vi "ecg_ncs_v1b.vi"() -> ()   [LabVIEW 2016]
uses:
  <instrlib>/niUSRP/niUSRP Timestamp.ctl
  C:/Program Files/National Instruments/LabVIEW 2016/examples/Instrument IO/Serial/support/Serial - Settings.ctl
  <vilib>/Analysis/coordinate.llb/Wrap Angle (array).vi
  <instrlib>/niUSRP/niUSRP Configure Time Start Trigger.vi
  <vilib>/Instr/_visa.llb/VISA Configure Serial Port (Instr).vi
  <instrlib>/niUSRP/niUSRP Write Tx Data (2D CDB).vi
  <instrlib>/niUSRP/niUSRP Fetch Rx Data (2D CDB).vi
  <vilib>/Analysis/3filter.llb/Butterworth Filter (DBL).vi
  <vilib>/measure/NI_MABase.lvlib
  <vilib>/Analysis/NI_AALBase.lvlib
  <vilib>/Analysis/NI_AALPro.lvlib
  <vilib>/Analysis/NI_AAL_Angle.lvlib
panel:
  out "Poor Sensor Quality: \nSensor off":bool
  out "Poor Sensor Quality: \nSensor on":bool
  out "Heart Rate 2":u16[](array[numeric])
  out "Stop Loop":bool
  out "Loop index":i32
  out "size(s)":i32
  in  "Read Count":u32=960
  out "return count":u32
  out "Serial Settings:Number of Bytes at Serial Port":u32
  in  "Serial Settings":T1={"baud rate"=57600, "data bits"=8, "parity"=enum."None", "stop bits"=10, "flow control"=0} {"flow control" items=["None"=0, "XON/XOFF"=1, "RTS/CTS"=2, "DTR/DSR"=4]; "stop bits" items=["1.0"=10, "1.5"=15, "2.0"=20]; "data bits" min=5 max=8 step=1; "baud rate" items=["75"=75, "110"=110, "134"=134, "150"=150, "300"=300, "600"=600, "1200"=1200, "1800"=1800, "2400"=2400, "4800"=4800, "7200"=7200, "9600"=9600, "14400"=14400, "19200"=19200, "28800"=28800, "38400"=38400, "56000"=56000, "57600"=57600, "115200"=115200, "128000"=128000, "230400"=230400]}
  in  "VISA resource name":refnum<visa-resource-name>="bmd101"
  in  "?":enum32{"ECG", "Heart Rate"}(tab)
  out "ECG":i16(graph)
  out "Heart Rate":u8[](graph)
  in  "Stop":bool
  in  "File Name":string="Test"
  in  "order1":i32=5
  in  "Path":path=path "D:/Research/SummerFall17Spring18/CnC/NCS/EcgNcsCorrelation"
  in  "Low-Pass Freq":dbl=200.0 format="%#_13g"
  in  "Sampling Rate":i32=500
  out "Gain":dbl=-15.0
  out "Bandwidth":dbl=56000000.0
  out "Coerced Carrier Frequency":dbl=2000000000.0 format="%#.17g"
  out "Coerced Tx IQ rate":dbl=1000000.0
  out "Coerced Rx IQ rate":dbl=1000000.0
  out "error IO":errorcluster={"status"=FALSE, "code"=-1074118647, "source"=""}
  in  "Rx Number of Samples":i32=20000
  in  "Tab Control 2":enum32{"NI-294x/295x", "NI-2900/2901"}(tab)=enum."NI-2900/2901"
  in  "channel 0 carrier\n frequency [Hz]":dbl=2000000000.0 format="%#_6p"
  in  "Rx carrier frequency [Hz]":dbl=2000000000.0 format="%#_6p"
  in  "Tx carrier frequency [Hz]":dbl=1000000000.0 format="%#_6p"
  in  "Start Trigger Time":T2={"whole seconds"=1, "fractional seconds"=0.0}
  out "Tx Active Antenna":string="TX1"
  in  "Tab Control":T3(tab)
  out "NCS tag Amp":dbl[](graph)=[0.013332788438327721, 0.0131552898712497, 0.012994905519721597, 0.012986271887777701, 0.013075284595455733, 0.013191204808537919, 0.013351894528100879, 0.01345386740636616, 0.013382234051438232, 0.013180163786137358]
  out "NCS tag Phase":dbl[](graph)=[114.08993023907641, 111.82225141412982, 110.02998222947944, 109.41153055749608, 110.12587965469353, 112.16042160734105, 113.81215100166591, 114.51260226782536, 113.6206368361215, 111.46787264294511]
  out "IQ":dbl[][](graph)
  out "Tag Amp":dbl[](graph)
  out "Tag Phase":dbl[](graph)
  out "Tx Waveform Graph":waveform(dbl)[](graph)=[{"t0"=timestamp(0 s since 1904-01-01), "dt"=1e-06, "Y"=array[2000 elements]}, {"t0"=timestamp(0 s since 1904-01-01), "dt"=1e-06, "Y"=array[2000 elements]}]
  in  "Channel 0\nTone Amplitude":dbl=0.707 step=0.05 format="%#.6g"
  in  "Channel 0 \nTone Frequency":dbl=5000.0 format="%#_6p"
  in  "Waveform Size":dbl=2000.0
  in  "Rx Active Antenna":string="RX2"
  in  "Device Name":refnum<k15>="MyB200"
  in  "Tx Gain":dbl=28.0 format="%#_6f"
  in  "Tx IQ Rate":dbl=1000000.0 format="%#_6p"
  in  "Rx Gain":dbl=32.0 format="%#_6f"
  in  "Rx IQ Rate":dbl=1000000.0 format="%#_6p"
  # "Rx Settings"
  # "Tx Settings"
  # "Note that on the NI-2900 and NI-2901, both Rx channels share an LO and both Tx channels share an LO. However, on the NI-294x/295x devices, Rx and Tx of channel 0 share an LO and Rx and Tx of channel 1 share an LO."
  # "This Tx graph should always have end and start tied up since this is being sent in a loop continuously. Otherwise phase jumps will be noticed."
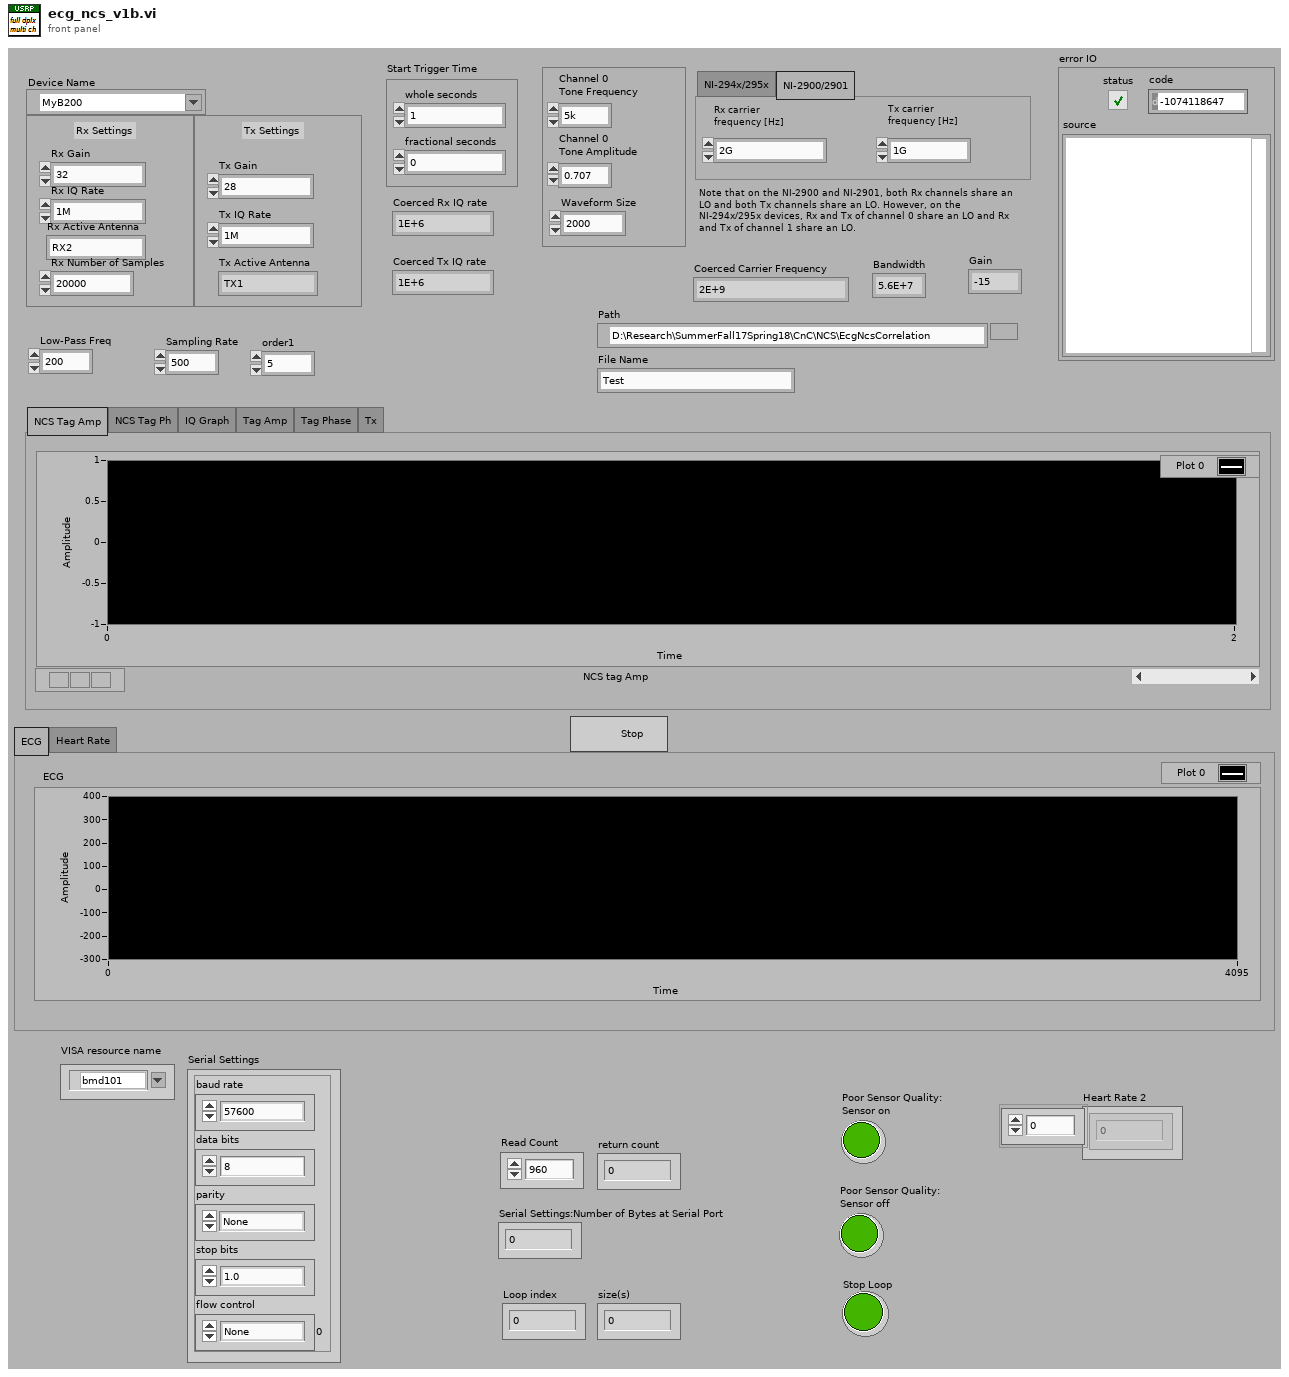
[diagram p1: front panel]
types:
  T1 = typedef "Serial - Settings.ctl" = cluster{"baud rate":u32, "data bits":u16, "parity":enum16{"None", "Odd", "Even", "Mark", "Space"}, "stop bits":u16, "flow control":u16}
  T2 = typedef "niUSRP Timestamp.ctl" = cluster{"whole seconds":u64, "fractional seconds":dbl}
  T3 = enum32{"NCS Tag Amp", "NCS Tag Ph", "IQ Graph", "Tag Amp", "Tag Phase", "Tx"}
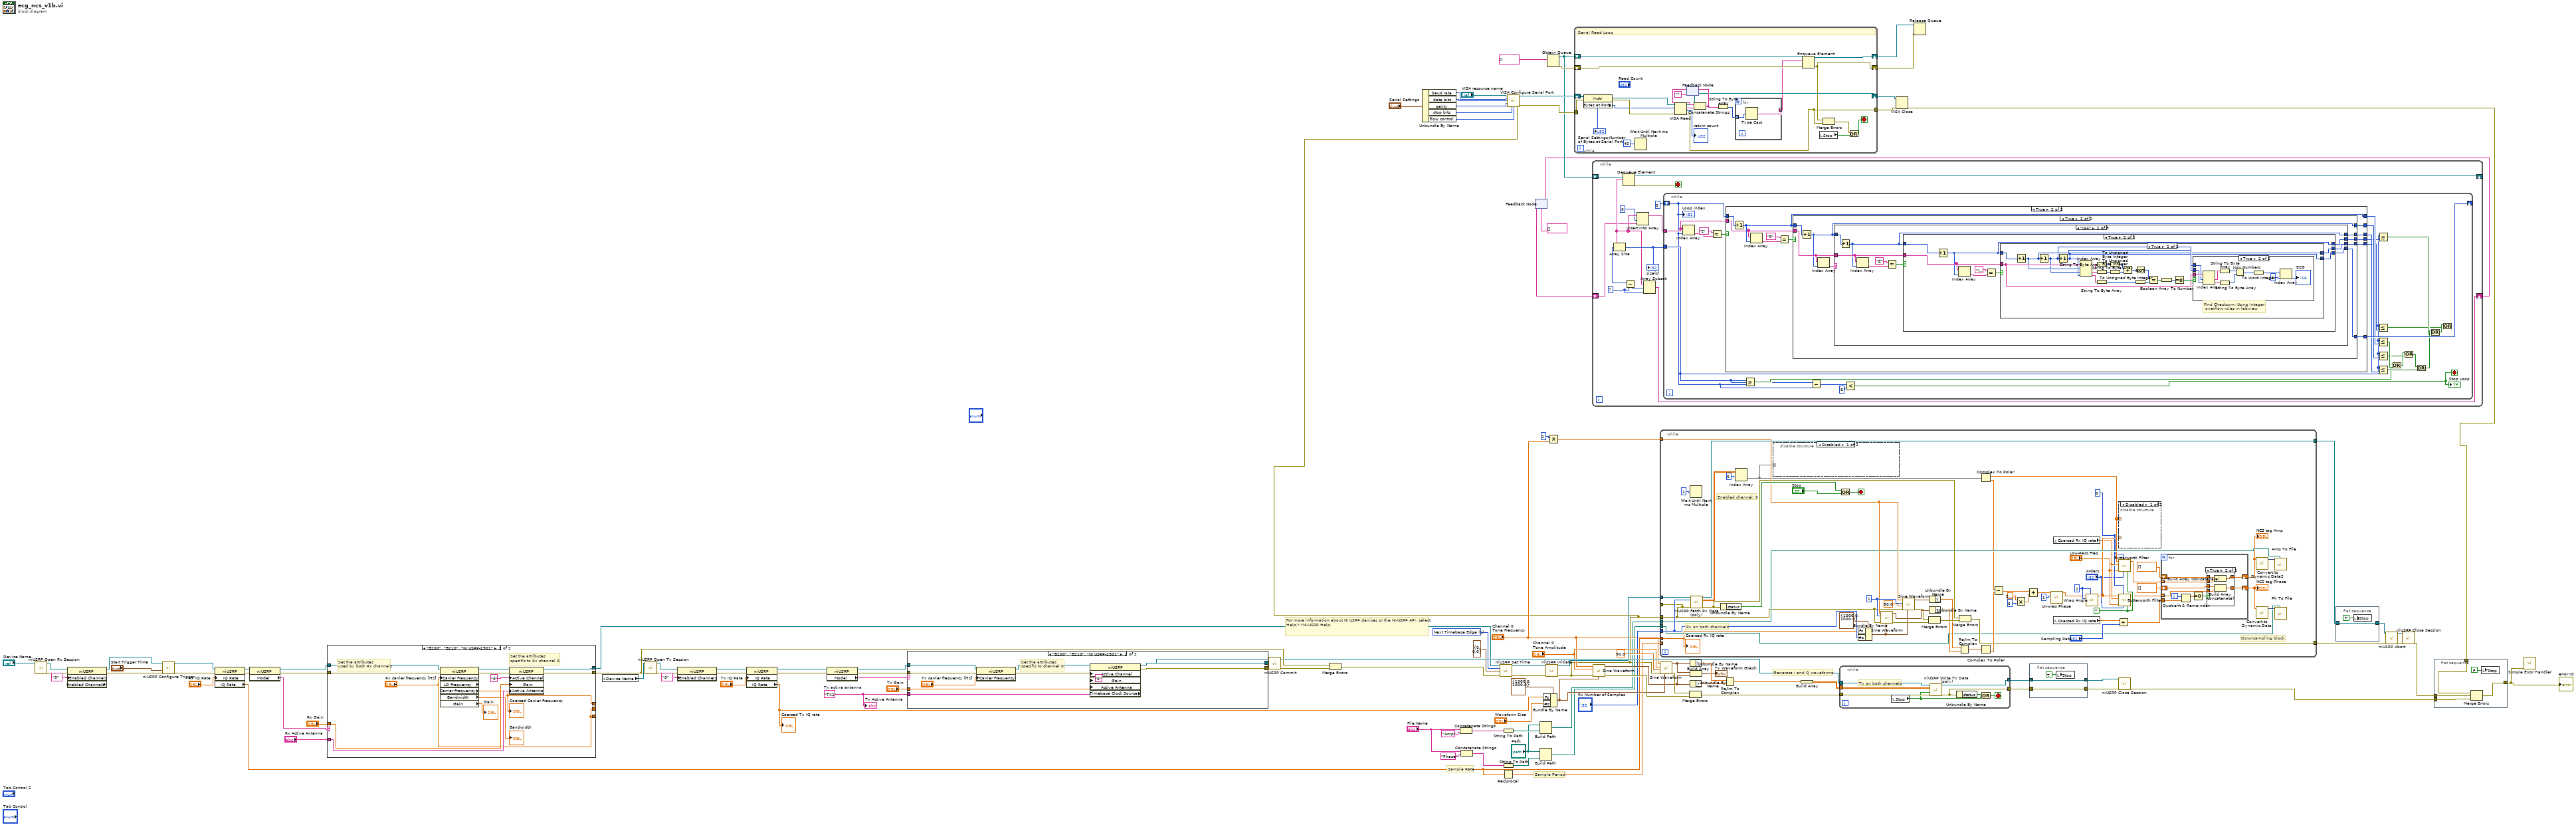
[diagram p0: block diagram]
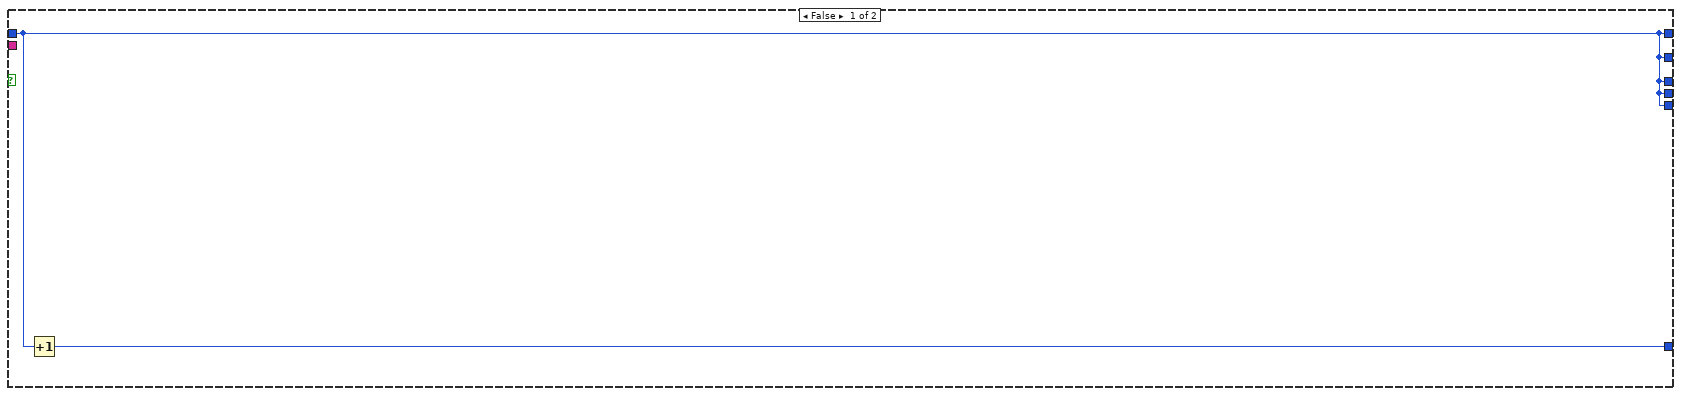
[diagram p2: hidden frame]
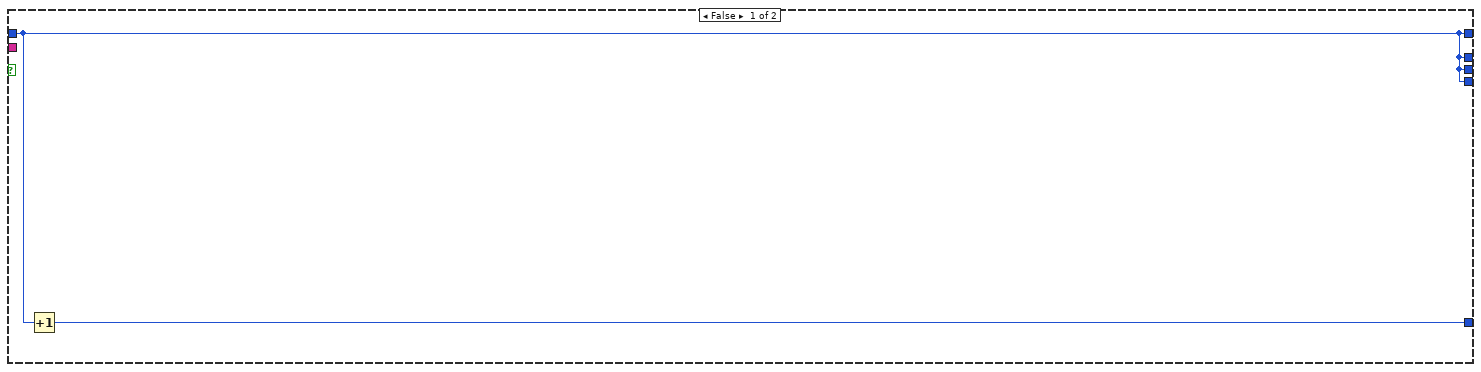
[diagram p3: hidden frame]
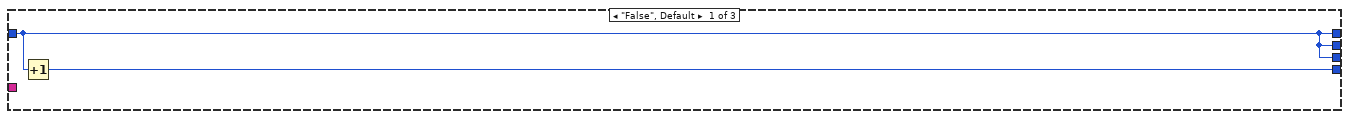
[diagram p4: hidden frame]
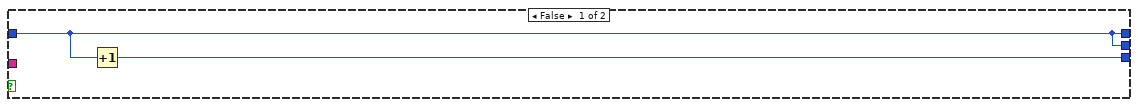
[diagram p5: hidden frame]
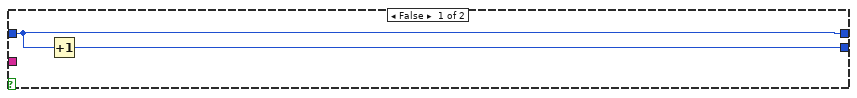
[diagram p6: hidden frame]
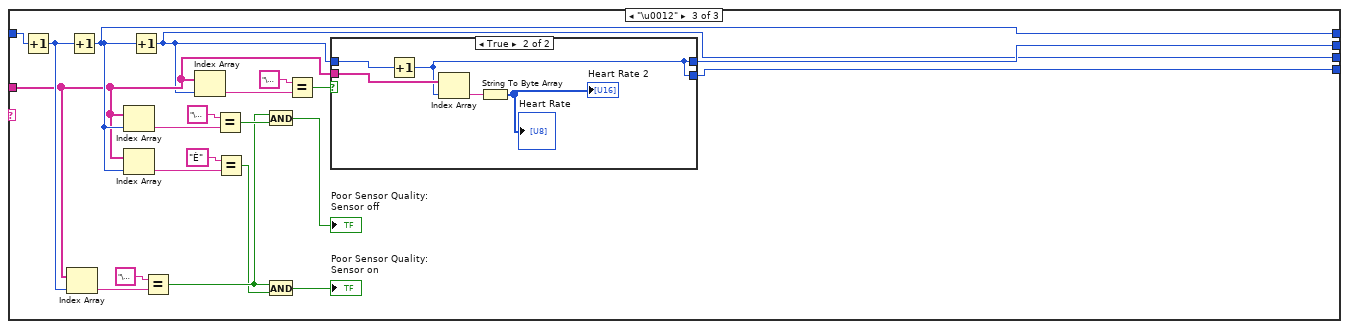
[diagram p8: hidden frame]
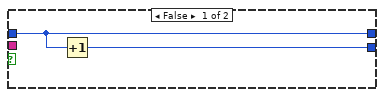
[diagram p9: hidden frame]
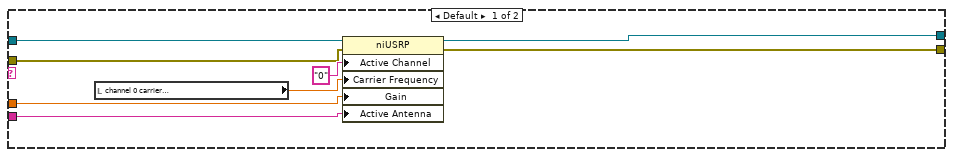
[diagram p10: hidden frame]
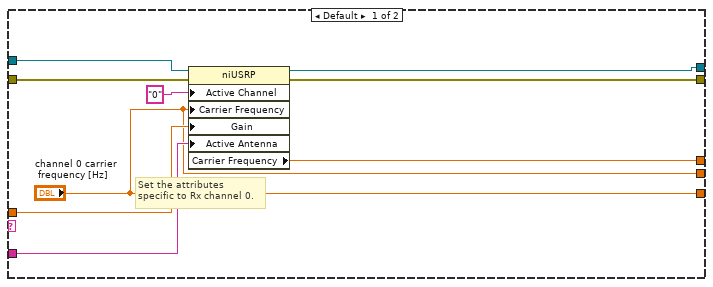
[diagram p11: hidden frame]
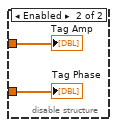
[diagram p12: hidden frame]
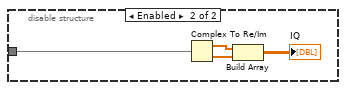
[diagram p13: hidden frame]
diagram:
  w81 = 1 items=["Now", "Next Timebase Edge"] ("apply timestamp")
  w50 = "TX1"  # Tx active antenna
  # "Sample Rate"
  # "Sample Period"
  # "For more information about NI USRP devices or the NI-USRP API, select Help>>NI-USRP Help."
  # "Generate I and Q waveforms."
  n1 = call <instrlib>:"niUSRP Open Rx Session.vi"("device names"="Device Name") -> ("session handle out"=w80:refnum<k15>, "error out"=w79:errorcluster)  [unwired: 13 in]
  n2 = property class="niUSRP" props=["Enabled Channels", "Enabled Channels"](reference=w80, error in=w79, "Enabled Channels"="0" ("Configuration:Enabled Channels")) -> (reference out=w78:refnum<k15>, error out=w77:errorcluster)  [unwired: 1 out]
  n3 = call-poly <instrlib>:"niUSRP Configure Trigger.vi"("session handle"=w78, "start trigger time"="Start Trigger Time", "error in (no error)"=w77) -> ("session handle out"=w74:refnum<k15>, "error out"=w73:errorcluster)  [unwired: 11 in]
  n4 = property class="niUSRP"(reference=w74, error in=w73, "IQ Rate"="Rx IQ Rate") -> (reference out=w70:refnum<k15>, error out=w71:errorcluster, "IQ Rate"=w37:dbl)
  n5 = property class="niUSRP"(reference=w70, error in=w71) -> (reference out=w65:refnum<k15>, error out=w66:errorcluster, "Model"=w67:string)
  n6 = case shown="\"B200\", \"B210\", \"NI USRP-2901\"" w67 {
    tunnel: w66 -> [w116 w126]
    tunnel: w65 -> [w115 w127]
    tunnel: [w112 w123] -> w69
    tunnel: [w111 w122] -> w68
    tunnel: "Rx Gain" -> [w114 w129]
    tunnel: "Rx Active Antenna" -> [w113 w128]
    tunnel: [w109 w118] -> _
    tunnel: ["channel 0 carrier\n frequency [Hz]" "Rx carrier frequency [Hz]"] -> _
    tunnel: ["channel 0 carrier\n frequency [Hz]" "Rx carrier frequency [Hz]"] -> _
    frame Default {
      # "Set the attributes \nspecific to Rx channel 0."
      n7 = property class="niUSRP"(reference=w115, error in=w116, "Active Channel"="0", "Carrier Frequency"="channel 0 carrier\n frequency [Hz]", "Gain"=w114, "Active Antenna"=w113) -> (reference out=w112:refnum<k15>, error out=w111:errorcluster, "Carrier Frequency"=w109:dbl)
    }
    frame "B200", "B210", "NI USRP-2901" {
      # "Set the attributes \nused by both Rx channels"
      # "Set the attributes \nspecific to Rx channel 0."
      n8 = property class="niUSRP" props=["Carrier Frequency", "LO Frequency", "Carrier Frequency", "Bandwidth", "Gain"](reference=w127, error in=w126, "Carrier Frequency"="Rx carrier frequency [Hz]") -> (reference out=w125:refnum<k15>, error out=w124:errorcluster, "Carrier Frequency"=w118:dbl, "Bandwidth"=→"Bandwidth":dbl, "Gain"=→"Gain":dbl)  [unwired: 1 out]
      "Coerced Carrier Frequency" <- w118
      n9 = property class="niUSRP"(reference=w125, error in=w124, "Active Channel"="0", "Gain"=w129, "Active Antenna"=w128) -> (reference out=w123:refnum<k15>, error out=w122:errorcluster)
    }
  }
  n10 = local read "Device Name"() -> (w102:refnum<k15>)
  n11 = call <instrlib>:"niUSRP Open Tx Session.vi"("device names"=w102, "error in (no error)"=w68) -> ("session handle out"=w76:refnum<k15>, "error out"=w75:errorcluster)  [unwired: 12 in]
  n12 = property class="niUSRP"(reference=w76, error in=w75, "Enabled Channels"="0" ("Configuration:Enabled Channels")) -> (reference out=w62:refnum<k15>, error out=w61:errorcluster)
  n13 = property class="niUSRP"(reference=w62, error in=w61, "IQ Rate"="Tx IQ Rate") -> (reference out=w56:refnum<k15>, error out=w57:errorcluster, "IQ Rate"=w54:dbl)
  "Coerced Tx IQ rate" <- w54
  n14 = property class="niUSRP"(reference=w56, error in=w57) -> (reference out=w58:refnum<k15>, error out=w59:errorcluster, "Model"=w55:string)
  n15 = case shown="\"B200\", \"B210\", \"NI USRP-2901\"" w55 {
    tunnel: "Tx Gain" -> [w138 w148]
    tunnel: w50 -> [w136 w146]
    tunnel: [w132 w140] -> w52
    tunnel: [w131 w139] -> w53
    tunnel: w59 -> [w135 w142]
    tunnel: w58 -> [w134 w145]
    frame Default {
      n16 = local read "channel 0 carrier\n frequency [Hz]"() -> (w133:dbl)
      n17 = property class="niUSRP"(reference=w134, error in=w135, "Active Channel"="0", "Carrier Frequency"=w133, "Gain"=w138, "Active Antenna"=w136) -> (reference out=w132:refnum<k15>, error out=w131:errorcluster)
    }
    frame "B200", "B210", "NI USRP-2901" {
      # "Set the attributes \nspecific to channel 0."
      n18 = property class="niUSRP"(reference=w145, error in=w142, "Carrier Frequency"="Tx carrier frequency [Hz]") -> (reference out=w144:refnum<k15>, error out=w143:errorcluster)
      n19 = property class="niUSRP" props=["Active Channel", "Gain", "Active Antenna", "Timebase Clock Source"](reference=w144, error in=w143, "Active Channel"="0", "Gain"=w148, "Active Antenna"=w146) -> (reference out=w140:refnum<k15>, error out=w139:errorcluster)  [unwired: 1 out]
    }
  }
  n20 = call <instrlib>:"niUSRP Commit.vi"("session handle"=w52, "error in (no error)"=w53) -> ("session handle out"=w104:refnum<k15>, "error out"=w105:errorcluster)  [unwired: 12 in]
  n21 = Merge Errors(w68, w105) -> (w83:errorcluster)
  n22 = Unbundle By Name("Serial Settings") -> ("baud rate"=w20:u32, "data bits"=w19:u16, "parity"=w18:enum16{"None", "Odd", "Even", "Mark", "Space"}, "stop bits"=w17:u16, "flow control"=w16:u16)
  n23 = Concatenate Strings("File Name", "Amp") -> (w30:string)
  n24 = Concatenate Strings("File Name", "Phase") -> (w26:string)
  n25 = call <instrlib>:"niUSRP Set Time.vi"("session handle"=w69, "apply timestamp"=w81, "timestamp"=T2 {"whole seconds"=0, "fractional seconds"=0.0}, "error in (no error)"=w83) -> ("session handle out"=w85:refnum<k15>, "error out"=w84:errorcluster)  [unwired: 10 in]
  n26 = String To Path(string=w30) -> (path=w29:path)
  n27 = String To Path(string=w26) -> (path=w25:path)
  n28 = Reciprocal(x=w37) -> (1/x=w88:dbl)
  n29 = feedback #1(string[] []) -> (w4:string[])
  n30 = Build Path(base path="Path", name or relative path=w29) -> (appended path=w32:path)
  n31 = Build Path(base path="Path", name or relative path=w25) -> (appended path=w23:path)
  n32 = Bundle By Name(cluster=cluster{"Fs":dbl, "#s":dbl} {"Fs"=1000.0, "#s"=1000.0} ("sampling info"), "Fs"=w54, "#s"="Waveform Size") -> (w87:cluster{"Fs":dbl, "#s":dbl})
  n33 = call <instrlib>:"niUSRP Initiate.vi"("session handle"=w85, "error in (no error)"=w84) -> ("session handle out"=w108:refnum<k15>, "error out"=w1:errorcluster)  [unwired: 12 in]
  n34 = call-poly "VISA Configure Serial Port"("VISA resource name"="VISA resource name", "baud rate (9600)"=w20, "data bits (8)"=w19, "parity (0:none)"=w18, "error in (no error)"=w1, "stop bits (10: 1 bit)"=w17, "flow control (0:none)"=w16) -> ("VISA resource name out"=w12:refnum<visa-resource-name>, "error out"=w11:errorcluster)  [unwired: 3 in, 4 out]
  n35 = Obtain Queue(element data type=string[] []) -> (queue out=w6:refnum<queue>, error out=w8:errorcluster)  [unwired: 4 in, 1 out]
  n36 = Multiply(x=2, y="Channel 0 \nTone Frequency") -> (x*y=w34:dbl)
  n37 = while {
    shift-right: [w163] -> w13
    shift-left: w12 -> [w154]
    tunnel: w11 -> [w152]
    tunnel: [w156] -> w14
    shift-right: [w157] -> w10
    shift-left: w8 -> [w161]
    shift-right: [w158] -> w7
    shift-left: w6 -> [w159]
    stop <- w170 stop-if-true
    # "Serial Read Loop"
    n38 = property class="Instr"(reference=w154, error in=w152) -> (reference out=w153:refnum<visa-resource-name>, error out=w151:errorcluster, "Bytes at Port"=w150:u32)
    "Serial Settings:Number of Bytes at Serial Port" <- w150
    n39 = Wait Until Next ms Multiple(millisecond multiple=u32 40 ("milliseconds to wait")) -> ()  [unwired: 1 out]
    n40 = VISA Read(VISA resource name=w153, byte count=w150, error in (no error)=w151) -> (VISA resource name out=w163:refnum<visa-resource-name>, read buffer=w168:string, return count=→"return count":u32, error out=w156:errorcluster)
    n41 = feedback #2("") -> (w167:string)
    n42 = Concatenate Strings(w167, w168) -> (w165:string)
    n43 = feedback-in #2(w165) -> ()
    n44 = String To Byte Array(string=w165) -> (unsigned byte array=w162:u8[])
    n45 = for {
      tunnel: w162 -> [w172] mode=indexing
      tunnel: [w171] -> w160 mode=indexing
      n46 = Type Cast(x=w172) -> (*(type *) &x=w171:string)  [unwired: 1 in]
    }
    n47 = Enqueue Element(queue=w159, element=w160, error in (no error)=w161) -> (queue out=w158:refnum<queue>, error out=w157:errorcluster)  [unwired: 1 in, 1 out]
    n48 = local read "Stop"() -> (w149:bool)
    n49 = Merge Errors(w157, w156) -> (w155:errorcluster)
    n50 = Or(x=w155, y=w149) -> (x .or. y?=w170:bool)
  }
  n51 = while {
    shift-right: [w182] -> _
    shift-left: w6 -> [w183]
    shift-right: [w175] -> w5
    shift-left: w4 -> [w173]
    stop <- w181 stop-if-true
    w178 = 7
    n52 = Dequeue Element(queue=w183) -> (queue out=w182:refnum<queue>, element=w176:string[], error out=w181:errorcluster)  [unwired: 2 in, 1 out]
    n53 = Array Size(array=w176) -> (size(s)=w180:i32)
    "size(s)" <- w180
    n54 = Subtract(x=w180, y=w178) -> (x-y=w179:i32)
    n55 = Insert Into Array(array=w176, index=0, new element=w173) -> (w177:string[])
    n56 = Array Subset(array=w176, index=w179, length=w178) -> (w175:string[])
    n57 = while {
      tunnel: w177 -> [w205]
      shift-right: [w209] -> _
      shift-left: 0 -> [w188]
      tunnel: w180 -> [w189]
      stop <- w185 stop-if-true
      n58 = Index Array(array=w205, index=w188) -> (element=w208:string)
      n59 = Equal?(x="ª", y=w208) -> (x = y?=w206:bool)
      n60 = case shown="True" w206 {
        tunnel: w188 -> [w210 w220]
        tunnel: [w211 w218] -> w209
        tunnel: w205 -> [_ w212]
        tunnel: [w210 w217] -> w204
        tunnel: [w210 w216] -> w202
        tunnel: [w210 w215] -> w199
        tunnel: [w210 w214] -> w196
        tunnel: [w210 w213] -> w193
        frame False {
          n61 = Increment(x=w210) -> (x+1=w211:i32)
        }
        frame True {
          n62 = Increment(x=w220) -> (x+1=w217:i32)
          n63 = Index Array(array=w212, index=w217) -> (element=w222:string)
          n64 = Equal?(x="ª", y=w222) -> (x = y?=w219:bool)
          n65 = case shown="True" w219 {
            tunnel: w217 -> [w223 w226]
            tunnel: [w224 w232] -> w218
            tunnel: w212 -> [_ w231]
            tunnel: [w223 w227] -> w216
            tunnel: [w223 w230] -> w215
            tunnel: [w223 w229] -> w214
            tunnel: [w223 w228] -> w213
            frame False {
              n66 = Increment(x=w223) -> (x+1=w224:i32)
            }
            frame True {
              n67 = Increment(x=w226) -> (x+1=w227:i32)
              n68 = Index Array(array=w231, index=w227) -> (element=w225:string)
              n69 = case shown="\"\\04\"" w225 {
                tunnel: w227 -> [w233 w240 w305]
                tunnel: [w234 w239 w287] -> w232
                tunnel: w231 -> [_ w238 w289]
                tunnel: [w233 w237 w291] -> w230
                tunnel: [w233 w236 w288] -> w229
                tunnel: [w233 w235 w286] -> w228
                frame "False", Default {
                  n70 = Increment(x=w233) -> (x+1=w234:i32)
                }
                frame "\u0004" {
                  n71 = Increment(x=w240) -> (x+1=w237:i32)
                  n72 = Index Array(array=w238, index=w237) -> (element=w241:string)
                  n73 = Equal?(x="€", y=w241) -> (x = y?=w242:bool)
                  n74 = case shown="True" w242 {
                    tunnel: w237 -> [w244 w250]
                    tunnel: [w245 w249] -> w239
                    tunnel: w238 -> [_ w248]
                    tunnel: [w244 w247] -> w236
                    tunnel: [w244 w246] -> w235
                    frame False {
                      n75 = Increment(x=w244) -> (x+1=w245:i32)
                    }
                    frame True {
                      n76 = Increment(x=w250) -> (x+1=w247:i32)
                      n77 = Index Array(array=w248, index=w247) -> (element=w251:string)
                      n78 = Equal?(x="\u0002", y=w251) -> (x = y?=w252:bool)
                      n79 = case shown="True" w252 {
                        tunnel: w247 -> [w254 w259]
                        tunnel: [w255 w256] -> w249
                        tunnel: w248 -> [_ w260]
                        tunnel: [w254 w256] -> w246
                        frame False {
                          n80 = Increment(x=w254) -> (x+1=w255:i32)
                        }
                        frame True {
                          # "Find Checksum: Using Integer\n overflow rules in labview"
                          n81 = Increment(x=w259) -> (x+1=w258:i32)
                          n82 = Increment(x=w258) -> (x+1=w257:i32)
                          n83 = Increment(x=w257) -> (x+1=w256:i32)
                          n84 = Index Array(array=w260, index #1=w258, index #2=w257, index #3=w256) -> (element #1=w274:string, element #2=w273:string, element #3=w267:string)
                          n85 = String To Byte Array(string=w274) -> (unsigned byte array=w272:u8[])
                          n86 = String To Byte Array(string=w273) -> (unsigned byte array=w271:u8[])
                          n87 = String To Byte Array(string=w267) -> (unsigned byte array=w266:u8[])
                          n88 = To Unsigned Byte Integer(number=w272) -> (unsigned 8bit integer=w270:u8[])
                          n89 = To Unsigned Byte Integer(number=w271) -> (unsigned 8bit integer=w269:u8[])
                          n90 = Add(x=w270, y=w269) -> (x+y=w268:u8[])
                          n91 = Not(x=w268) -> (.not. x?=w265:u8[])
                          n92 = To Unsigned Byte Integer(number=w266) -> (unsigned 8bit integer=w264:u8[])
                          n93 = Equal?(x=w265, y=w264) -> (x = y?=w263:bool[])
                          n94 = Boolean Array To Number(Boolean array=w263) -> (number=w262:u32)
                          n95 = Equal To 0?(x=w262) -> (x = 0?=w261:bool)
                          n96 = case shown="True" w261 {
                            tunnel: w260 -> [_ w285]
                            tunnel: w258 -> [_ w279]
                            tunnel: w257 -> [_ w278]
                            frame False {
                            }
                            frame True {
                              n97 = Index Array(array=w285, index #1=w279, index #2=w278) -> (element #1=w284:string, element #2=w283:string)
                              n98 = String To Byte Array(string=w284) -> (unsigned byte array=w282:u8[])
                              n99 = String To Byte Array(string=w283) -> (unsigned byte array=w281:u8[])
                              n100 = Join Numbers(hi=w282, lo=w281) -> ((hi.lo)=w280:u16[])
                              n101 = To Word Integer(number=w280) -> (16bit integer=w277:i16[])
                              n102 = Index Array(array=w277, index=0) -> (element=→"ECG":i16)
                            }
                          }
                        }
                      }
                    }
                  }
                }
                frame "\u0012" {
                  n103 = Increment(x=w305) -> (x+1=w301:i32)
                  n104 = Index Array(array=w289, index=w301) -> (element=w304:string)
                  n105 = Increment(x=w301) -> (x+1=w291:i32)
                  n106 = Index Array(array=w289, index=w291) -> (element=w302:string)
                  n107 = Index Array(array=w289, index=w291) -> (element=w299:string)
                  n108 = Increment(x=w291) -> (x+1=w286:i32)
                  n109 = Equal?(x="\u0002", y=w304) -> (x = y?=w296:bool)
                  n110 = Index Array(array=w289, index=w286) -> (element=w292:string)
                  n111 = Equal?(x="\u0000", y=w302) -> (x = y?=w298:bool)
                  n112 = Equal?(x="È", y=w299) -> (x = y?=w295:bool)
                  n113 = And(x=w296, y=w298) -> (x .and. y?=→"Poor Sensor Quality: \nSensor off":bool)
                  n114 = And(x=w296, y=w295) -> (x .and. y?=→"Poor Sensor Quality: \nSensor on":bool)
                  n115 = Equal?(x="\u0003", y=w292) -> (x = y?=w290:bool)
                  n116 = case shown="True" w290 {
                    tunnel: w286 -> [w307 w313]
                    tunnel: w289 -> [_ w312]
                    tunnel: [w307 w311] -> w288
                    tunnel: [w308 w311] -> w287
                    frame False {
                      n117 = Increment(x=w307) -> (x+1=w308:i32)
                    }
                    frame True {
                      n118 = Increment(x=w313) -> (x+1=w311:i32)
                      n119 = Index Array(array=w312, index=w311) -> (element=w310:string)
                      n120 = String To Byte Array(string=w310) -> (unsigned byte array=→"Heart Rate 2" →"Heart Rate":u8[])
                    }
                  }
                }
              }
            }
          }
        }
      }
      n121 = Less Or Equal?(x=w189, y=w188) -> (x <= y?=w190:bool)
      n122 = Subtract(x=w189, y=w188) -> (x-y=w187:i32)
      n123 = Less?(x=w187, y=6) -> (x < y?=w185:bool)
      "Stop Loop" <- w185
      n124 = Less Or Equal?(x=w189, y=w196) -> (x <= y?=w194:bool)
      n125 = Less Or Equal?(x=w189, y=w193) -> (x <= y?=w191:bool)
      n126 = Less Or Equal?(x=w189, y=w204) -> (x <= y?=w203:bool)
      n127 = Less Or Equal?(x=w189, y=w202) -> (x <= y?=w200:bool)
      n128 = Less Or Equal?(x=w189, y=w199) -> (x <= y?=w197:bool)
      n129 = Or(x=w190, y=w203) -> (x .or. y?=w201:bool)
      n130 = Or(x=w201, y=w200) -> (x .or. y?=w198:bool)
      n131 = Or(x=w198, y=w197) -> (x .or. y?=w195:bool)
      n132 = Or(x=w195, y=w194) -> (x .or. y?=w192:bool)
      n133 = Or(x=w192, y=w191) -> ()  [unwired: 1 out]
      "Loop index" <- w188
    }
  }
  n134 = feedback-in #1(w5) -> ()
  n135 = call <vilib>:"Sine Waveform.vi"("sampling info"=w87, "error in (no error)"=w1, "amplitude"="Channel 0\nTone Amplitude", "frequency"="Channel 0 \nTone Frequency") -> ("error out"=w49:errorcluster, "signal out"=w97:waveform(dbl))  [unwired: 6 in]
  n136 = while {
    tunnel: w108 -> [w370]
    tunnel: w1 -> [w315]
    tunnel: [w369] -> w43
    tunnel: w88 -> [_]
    tunnel: "Rx Number of Samples" -> [w365]
    tunnel: w37 -> [w356]
    tunnel: w34 -> [w357]
    tunnel: [w346] -> w33
    tunnel: w32 -> [w345]
    tunnel: w23 -> [w320]
    tunnel: [w315] -> _
    stop <- w347 stop-if-true
    w332 = 2 ("y")
    w325 = TRUE
    w327 = 0
    w363 = 1
    # "Downsampling block"
    # "Enabled channel: 0"
    # "Rx on both channels"
    n137 = Wait Until Next ms Multiple(millisecond multiple=u32 1 ("milliseconds to wait")) -> ()  [unwired: 1 out]
    n138 = call-poly <instrlib>:"niUSRP Fetch Rx Data (poly).vi"("session handle"=w370, "number of samples"=w365, "error in (no error)"=w315) -> ("session handle out"=w369:refnum<k15>, "data"=w354:cdb[][], "error out"=w351:errorcluster)  [unwired: 9 in, 1 out]
    n139 = Unbundle By Name(w351) -> ("status"=w368:bool)
    n140 = Index Array(array=w354, index (row)=0 ("y")) -> (element=w353:cdb[])  [unwired: 1 in]
    n141 = disable-structure shown="Disabled" {
      disable-tunnel: w353 -> [_ w373]
      frame Disabled {
      }
      frame Enabled {
        n142 = Complex To Re/Im(x + iy=w373) -> (x=w376:dbl[], y=w375:dbl[])
        n143 = Build Array(w376, w375) -> (→"IQ":dbl[][])
      }
    }
    n144 = Or(x=w368, y="Stop") -> (x .or. y?=w347:bool)
    n145 = Bundle By Name(cluster=cluster{"Fs":dbl, "#s":dbl} {"Fs"=1000.0, "#s"=1000.0} ("sampling info"), "Fs"=w356, "#s"=w365) -> (w362:cluster{"Fs":dbl, "#s":dbl})
    n146 = call <vilib>:"Sine Waveform.vi"("sampling info"=w362, "error in (no error)"=w315, "amplitude"=w363, "frequency"=w357) -> ("error out"=w361:errorcluster, "signal out"=w366:waveform(dbl))  [unwired: 6 in]
    n147 = call <vilib>:"Sine Waveform.vi"("sampling info"=w362, "error in (no error)"=w315, "phase"=90.0, "amplitude"=w363, "frequency"=w357) -> ("error out"=w360:errorcluster, "signal out"=w358:waveform(dbl))  [unwired: 5 in]
    n148 = Merge Errors(w360, w361) -> (w359:errorcluster)
    n149 = Unbundle By Name(w358) -> ("Y"=w342:dbl[])
    n150 = Unbundle By Name(w366) -> ("Y"=w341:dbl[])
    n151 = Re/Im To Complex(1:w341, 2:w342) -> (0:w335:cdb[])
    n152 = Merge Errors(w351, w359) -> (w346:errorcluster)
    n153 = Complex To Polar(r * e^(i*theta)=w353) -> (r=w344:dbl[], theta=w330:dbl[])
    n154 = Complex To Polar(r * e^(i*theta)=w335) -> (theta=w336:dbl[])  [unwired: 1 out]
    n155 = Subtract(x=w330, y=w336) -> (x-y=w334:dbl[])
    n156 = Multiply(x=3.141592653589793, y=6) -> (x*y=w337:dbl)
    n157 = Add(x=w334, y=w337) -> (x+y=w333:dbl[])
    n158 = call <vilib>:"Unwrap Phase.vi"("phase unit"=1 ("y"), "Phase"=w333) -> ("Unwrapped Phase"=w331:dbl[])  [unwired: 8 in, 1 out]
    n159 = local read "Coerced Rx IQ rate"() -> (w328:dbl)
    n160 = local read "Coerced Rx IQ rate"() -> (w350:dbl)
    n161 = call-poly <vilib>:"Wrap Angle.vi"("angle units"=w332, "angle range"=w332, "Angle In"=w331) -> ("Angle Out"=w329:dbl[])  [unwired: 7 in, 1 out]
    n162 = Divide(x=w350, y="Sampling Rate") -> (x/y=w348:dbl)
    n163 = disable-structure shown="Disabled" {
      disable-tunnel: w344 -> [_ w372]
      disable-tunnel: w329 -> [_ w371]
      frame Disabled {
      }
      frame Enabled {
        "Tag Amp" <- w372
        "Tag Phase" <- w371
      }
    }
    n164 = call-poly <vilib>:"Butterworth Filter.vi"("init/cont (init:F)"=w325, "order"="order1", "filter type"=w327, "low cutoff freq: fl"="Low-Pass Freq", "sampling freq: fs"=w328, "X"=w344) -> ("Filtered X"=w343:dbl[])  [unwired: 2 in, 1 out]
    n165 = call-poly <vilib>:"Butterworth Filter.vi"("init/cont (init:F)"=w325, "order"="order1", "filter type"=w327, "low cutoff freq: fl"="Low-Pass Freq", "sampling freq: fs"=w328, "X"=w329) -> ("Filtered X"=w323:dbl[])  [unwired: 2 in, 1 out]
    n166 = for {
      tunnel: w343 -> [w386] mode=indexing
      shift-right: [w384] -> w318
      shift-left: dbl[] [] -> [w385]
      tunnel: w348 -> [w380]
      shift-right: [w378] -> w321
      shift-left: dbl[] [] -> [w379]
      tunnel: w323 -> [w377] mode=indexing
      i -> [w383]
      n167 = Quotient & Remainder(x=w383, y=w380) -> (x-y*floor(x/y)=w381:dbl)  [unwired: 1 out]
      n168 = Equal To 0?(x=w381) -> (x = 0?=w382:bool)
      n169 = case shown="True" w382 {
        tunnel: w386 -> [_ w394]
        tunnel: w385 -> [w388 w393]
        tunnel: [w388 w392] -> w384
        tunnel: w379 -> [w387 w391]
        tunnel: [w387 w390] -> w378
        tunnel: w377 -> [_ w389]
        frame False {
        }
        frame True {
          n170 = Build Array (concatenate)(w393, w394) -> (w392:dbl[])
          n171 = Build Array (concatenate)(w391, w389) -> (w390:dbl[])
        }
      }
    }
    "NCS tag Amp" <- w318
    "NCS tag Phase" <- w321
    n172 = call "Convert to Dynamic Data2"("Array"=w318) -> ("Dynamic Data Type"=w317:dynamicdata)  [unwired: 3 in]
    n173 = call "Convert to Dynamic Data"("Array"=w321) -> ("Dynamic Data Type"=w322:dynamicdata)  [unwired: 3 in]
    n174 = call "Amp To File"("Signals"=w317, "Filename"=w345) -> ()  [unwired: 15 in, 3 out]
    n175 = call "Ph To File"("Signals"=w322, "Filename"=w320) -> ()  [unwired: 15 in, 3 out]
    "Coerced Rx IQ rate" <- w356
  }
  n176 = call <vilib>:"Sine Waveform.vi"("sampling info"=w87, "error in (no error)"=w1, "phase"=90.0, "amplitude"="Channel 0\nTone Amplitude", "frequency"="Channel 0 \nTone Frequency") -> ("error out"=w48:errorcluster, "signal out"=w96:waveform(dbl))  [unwired: 5 in]
  n177 = Merge Errors(w48, w49) -> (w47:errorcluster)
  n178 = Unbundle By Name(w96) -> ("Y"=w95:dbl[])
  n179 = Build Array(w96, w97) -> (→"Tx Waveform Graph":waveform(dbl)[])
  n180 = Unbundle By Name(w97) -> ("Y"=w94:dbl[])
  n181 = Re/Im To Complex(1:w94, 2:w95) -> (0:w90:cdb[])
  n182 = Build Array(w90) -> (w89:cdb[][])
  n183 = while {
    tunnel: w104 -> [w402]
    tunnel: w47 -> [w401]
    tunnel: [w399] -> w46
    tunnel: [w397] -> w41
    tunnel: w89 -> [w396]
    stop <- w398 stop-if-true
    # "Tx on both channels"
    n184 = local read "Stop"() -> (w395:bool)
    n185 = call-poly <instrlib>:"niUSRP Write Tx Data (poly).vi"("session handle"=w402, "data"=w396, "end of data?"=w395, "error in (no error)"=w401) -> ("session handle out"=w397:refnum<k15>, "error out"=w399:errorcluster)  [unwired: 10 in]
    n186 = Unbundle By Name(w399) -> ("status"=w400:bool)
    n187 = Compound Arithmetic op=OR(w400, w395) -> (w398:bool)
  }
  n188 = VISA Close(VISA resource name=w13, error in (no error)=w14) -> (error out=w2:errorcluster)
  n189 = Release Queue(queue=w7, error in (no error)=w10) -> ()  [unwired: 1 in, 3 out]
  n190 = flat-sequence {
    tunnel: [w404] -> w45
    tunnel: w46 -> [w404]
    tunnel: [w403] -> w42
    tunnel: w41 -> [w403]
    frame #0 {
      n191 = local write "Stop"(TRUE ("STOP")) -> ()
    }
  }
  n192 = call <instrlib>:"niUSRP Close Session.vi"("session handle"=w42, "error in (no error)"=w45) -> ("error out"=w40:errorcluster)  [unwired: 13 in]
  n193 = flat-sequence {
    tunnel: [w406] -> w44
    tunnel: w43 -> [w406]
    frame #0 {
      n194 = local write "Stop"(TRUE ("STOP")) -> ()
    }
  }
  n195 = call <instrlib>:"niUSRP Abort.vi"("session handle"=w44, "error in (no error)"=w33) -> ("session handle out"=w101:refnum<k15>, "error out"=w100:errorcluster)  [unwired: 12 in]
  n196 = call <instrlib>:"niUSRP Close Session.vi"("session handle"=w101, "error in (no error)"=w100) -> ("error out"=w38:errorcluster)  [unwired: 13 in]
  n197 = flat-sequence {
    tunnel: w40 -> [w411]
    tunnel: [w410] -> w22
    tunnel: w38 -> [w409]
    tunnel: w2 -> [w408]
    frame #0 {
      n198 = Merge Errors(w408, w409, w411) -> (w410:errorcluster)
      n199 = local write "Stop"(FALSE ("STOP")) -> ()
    }
  }
  n200 = call <vilib>:"Simple Error Handler.vi"("error in (no error)"=w22) -> ()  [unwired: 1 in, 8 out]
  "Tx Active Antenna" <- w50
  "error IO" <- w22
